vi "Send Mute Single.vi"(7 "Message Priority (Normal)":T1=enum."Normal", 8 "error in (no error)":errorcluster, 9 "Mute":bool, 10 "Detector":u8, 11 "Message Enqueuer":refnum<class "Message Enqueuer.lvclass">) -> (0 "error out":errorcluster, 3 "Message Enqueuer out":refnum<class "Message Enqueuer.lvclass">)   [LabVIEW 2015, in "KIT-QVA.lvlib" / "Mute Single Msg.lvclass"]
doc: "Sends the <B>KIT-QVA.lvlib:Mute Single Msg.lvclass</B> message.\n\n<B>KIT-QVA.lvlib:KIT-QVA.lvclass:Mute Single.vi</B> Description:\n\nActivate or deactivate time unlimited muting of selected detector."
uses:
  Mute Single Msg.lvclass
  <vilib>/ActorFramework/Message Enqueuer/Message Enqueuer.lvclass
  <vilib>/ActorFramework/Message Enqueuer/Message Priority.ctl
  Mute Single Msg.lvclass/Mute Single Msg.ctl
  <vilib>/ActorFramework/Message Enqueuer/Message Enqueuer.lvclass/Message Enqueuer.ctl
  <vilib>/ActorFramework/Message Priority Queue/Priority Enqueue.vi
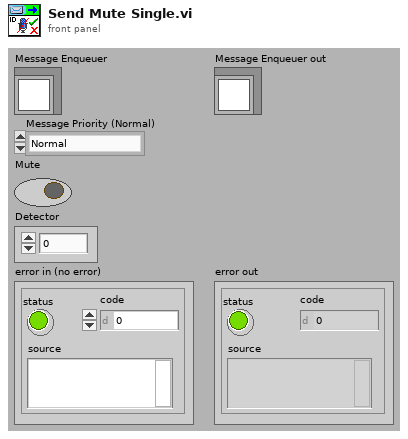
[diagram p1: front panel]
types:
  T1 = typedef "Actor Framework.lvlib/Message Enqueuer.lvclass/Message Priority.ctl" = enum16{"Low", "Normal", "High"}
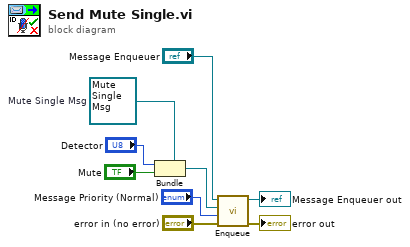
[diagram p0: block diagram]
diagram:
  w3 = refnum<class "Mute Single Msg.lvclass"> refnum  # Mute Single Msg
  n1 = Bundle(cluster=w3, "Detector", "Mute") -> (w6:refnum<class "Mute Single Msg.lvclass">)
  n2 = call <vilib>:"Enqueue.vi"("error in (no error)"="error in (no error)", "Message Priority (Normal)"="Message Priority (Normal)", "Message"=w6, "Message Enqueuer in"="Message Enqueuer") -> ("error out"=→"error out":errorcluster, "Message Enqueuer out"=→"Message Enqueuer out":refnum<class "Message Enqueuer.lvclass">)  [unwired: 6 in]
